vi "ROI entry-Get last ROI ID.vi"(8 "error in (no error)":errorcluster) -> (0 "error out":errorcluster, 1 "NO ROI":bool, 2 "ROI ID":i32, 3 "ROI ID Enum":T1)   [LabVIEW 2013]
uses:
  Typedefs/ROI ID Enum.ctl
  Typedefs/ROI management FG states.ctl
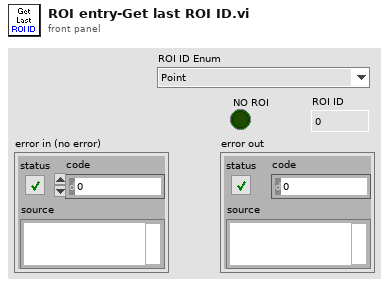
[diagram p1: front panel]
types:
  T1 = typedef "ROI ID Enum.ctl" = enum16{"Point", "MiniScan", "Comp. MiniScan", "Rectangle", "Comp. volume", "Arb. plane point"}
  T2 = typedef "ROI management FG states.ctl" = enum16{"Read", "Write", "Clear Last", "Clear All", "Update ROIs time", "Reload last ROI set", "Offset all ROI", "Offset visible ROI"}
  T3 = typedef "ROI parameters data type.ctl" = cluster{"ROI index":dbl, "ROI ID":dbl, "ROI Time (ns)":dbl, "Pixels in ROI":dbl, "X start":dbl, "Y start":dbl, "Z start":dbl, "X stop":dbl, "Y stop":dbl, "Z stop":dbl, "Angle (deg)":dbl, "Composite ID":dbl, "Number of lines":dbl, "Frame Size":dbl, "Zoom":dbl, "Laser Power (%)":dbl, "ROI group ID":dbl}
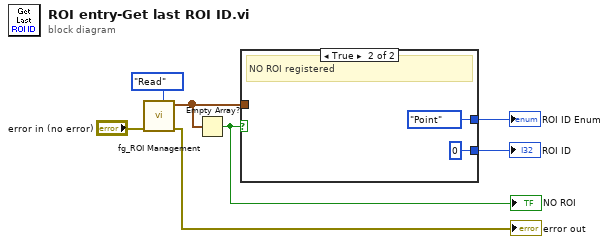
[diagram p0: block diagram]
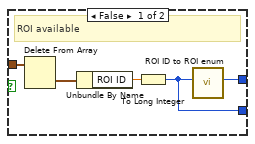
[diagram p2: hidden frame]
diagram:
  n1 = call "fg_ROI Management.vi"("Function"=ROI_management_FG_states."Read", "error in (no error)"="error in (no error)") -> ("error out"=→"error out":errorcluster, "ROI Setup"=w4:T3[])  [unwired: 5 in, 3 out]
  n2 = Empty Array?(array=w4) -> (empty?=w3:bool)
  "NO ROI" <- w3
  n3 = case shown="True" w3 {
    tunnel: [w12 ROI_ID_Enum."Point" ("ROI Enum")] -> w7
    tunnel: [w9 0] -> w5
    tunnel: w4 -> [w8 _]
    frame False {
      # "ROI available"
      n4 = Delete From Array(array=w8) -> (deleted portion=w10:T3)  [unwired: 2 in, 1 out]
      n5 = Unbundle By Name(w10) -> ("ROI ID"=w11:dbl)
      n6 = To Long Integer(number=w11) -> (32bit integer=w9:i32)
      n7 = call "ROI ID to ROI enum.vi"("ROI ID"=w9) -> ("ROI Enum"=w12:T1)  [unwired: 6 in]
    }
    frame True {
      # "NO ROI registered"
    }
  }
  "ROI ID Enum" <- w7
  "ROI ID" <- w5
